vi "Write Call request.vi"(8 "error in (no error)":errorcluster, 10 "Cluster":T1, 11 "CallRequest (MsgPack) in":refnum<class "CallRequest (MsgPack).lvclass">) -> (0 "error out":errorcluster, 3 "CallRequest (MsgPack) out":refnum<class "CallRequest (MsgPack).lvclass">)   [LabVIEW 2020, in "wamplv.lvlib" / "CallRequest (MsgPack).lvclass"]
uses:
  CallRequest (MsgPack).lvclass
  TypeDefs/CALL request (MsgPack).ctl
  MessagePack/MsgPackArray/MsgPackArray.lvclass
  MessagePack/MsgPackMap/MsgPackMap.lvclass
  WAMP Client/API/TypeDefs/RESULT payload (MsgPack).ctl
  WAMP Client/API/TypeDefs/Combined error.ctl
  WAMP Client/API/TypeDefs/WAMP error.ctl
  CallRequest (MsgPack).lvclass/CallRequest (MsgPack).ctl
  WAMP Client/WAMP Client.lvclass
  wamplv.lvlib
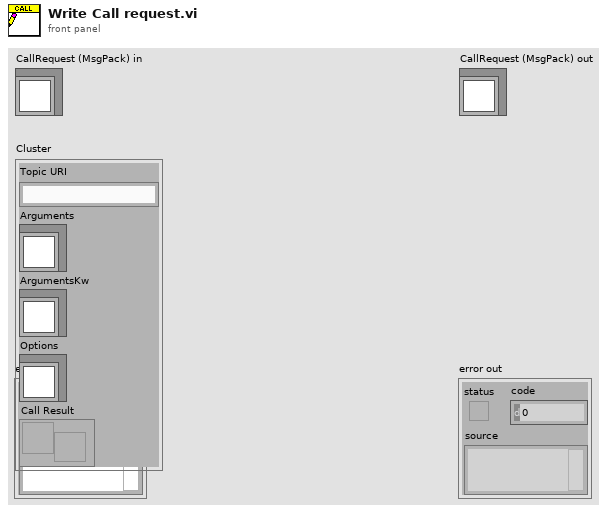
[diagram p1: front panel]
types:
  T1 = typedef "wamplv.lvlib/CALL request (MsgPack).ctl" = cluster{"Topic URI":string, "Arguments":refnum<class "MsgPackArray.lvclass">, "ArgumentsKw":refnum<class "MsgPackMap.lvclass">, "Options":refnum<class "MsgPackMap.lvclass">, "Call Result":refnum<notifier>}
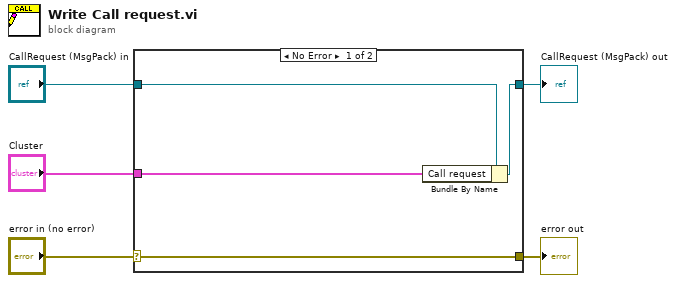
[diagram p0: block diagram]
diagram:
  n1 = case shown="No Error" "error in (no error)" {
    selector: "error in (no error)" -> [w9 w10]
    tunnel: [w9 w10] -> w4
    tunnel: [w7 w11] -> w2
    tunnel: "CallRequest (MsgPack) in" -> [w8 w11]
    tunnel: "Cluster" -> [w6 _]
    frame No Error {
      n2 = Bundle By Name(cluster=w8, "Call request"=w6) -> (w7:refnum<class "CallRequest (MsgPack).lvclass">)
    }
    frame Error {
    }
  }
  "error out" <- w4
  "CallRequest (MsgPack) out" <- w2
